vi "write_data.vi"(8 "error in (no error)":errorcluster, 10 "data":T1, 11 "KMeans in":refnum<class "KMeans.lvclass">) -> (0 "error out":errorcluster, 3 "KMeans out":refnum<class "KMeans.lvclass">)   [LabVIEW 2020, in "KMeans.lvclass"]
uses:
  KMeans.lvclass
  Controls/kmeans_data.ctl
  KMeans.lvclass/KMeans.ctl
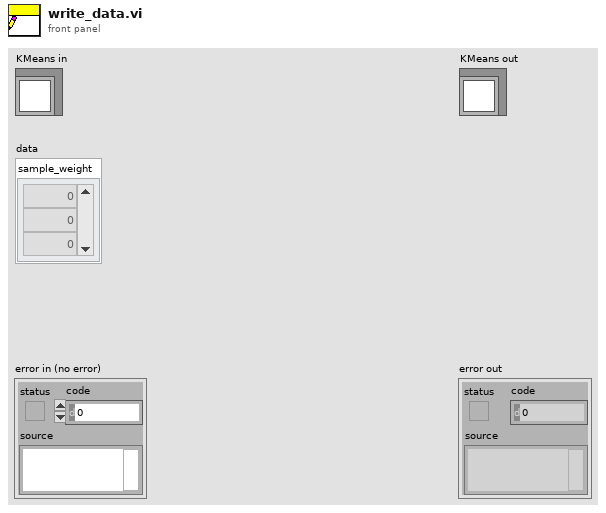
[diagram p1: front panel]
types:
  T1 = typedef "kmeans_data.ctl" = cluster{"sample_weight":dbl[]}
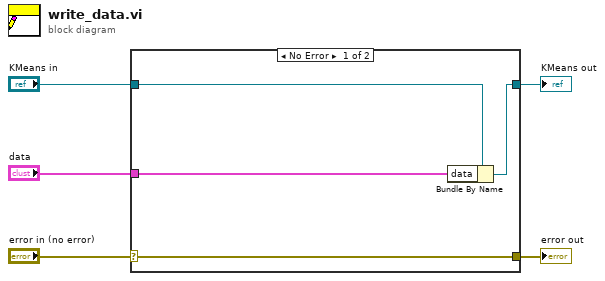
[diagram p0: block diagram]
diagram:
  n1 = case shown="No Error" "error in (no error)" {
    selector: "error in (no error)" -> [w9 w10]
    tunnel: [w9 w10] -> w4
    tunnel: [w7 w11] -> w2
    tunnel: "KMeans in" -> [w8 w11]
    tunnel: "data" -> [w6 _]
    frame No Error {
      n2 = Bundle By Name(cluster=w8, "data"=w6) -> (w7:refnum<class "KMeans.lvclass">)
    }
    frame Error {
    }
  }
  "error out" <- w4
  "KMeans out" <- w2
